vi "Constants.vi"() -> ()   [LabVIEW 2014, in "CAN Bus Monitor Shared.lvlib"]
doc: "Use this Global VI to access the GUIDs assigned to the page resources of the Custom Device."
uses:
  CAN Bus Monitor Shared.lvlib
panel:
  in  "Tab Control":enum32{"GUIDS", "Constants", "Properties"}(tab)=enum."Constants"
  in  "CAN Bus Monitor":string="f129a45f-35ad-474e-bc0d-2bc21d55f23c"
  in  "Baud Rate":string="Baud Rate"
  in  "Port Name":string="Port Name"
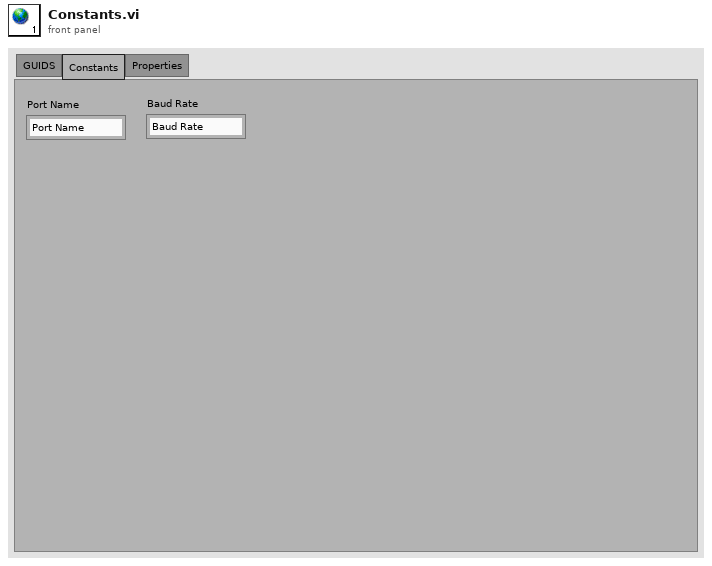
[diagram p1: front panel]
diagram:
